vi "InitPos.vi"(8 "error in (no error)":errorcluster caption="错误输入（无错误）", 11 "RandomMoveBool 输入":refnum<class "RandomMoveBool.lvclass">) -> (0 "error out":errorcluster caption="错误输出", 3 "RandomMoveBool 输出":refnum<class "RandomMoveBool.lvclass">)   [LabVIEW 2018, in "RandomMoveBool.lvclass"]
uses:
  RandomMoveBool.lvclass
  <vilib>/Utility/miscctls.llb/LVPositionTypeDef.ctl
  RandomMoveBool.lvclass/RandomMoveBool.ctl
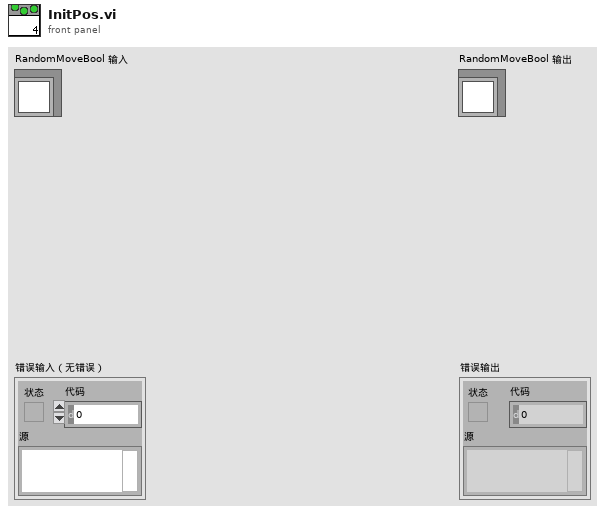
[diagram p1: front panel]
types:
  T1 = typedef "LVPositionTypeDef.ctl" = cluster{"Left":i32, "Top":i32}
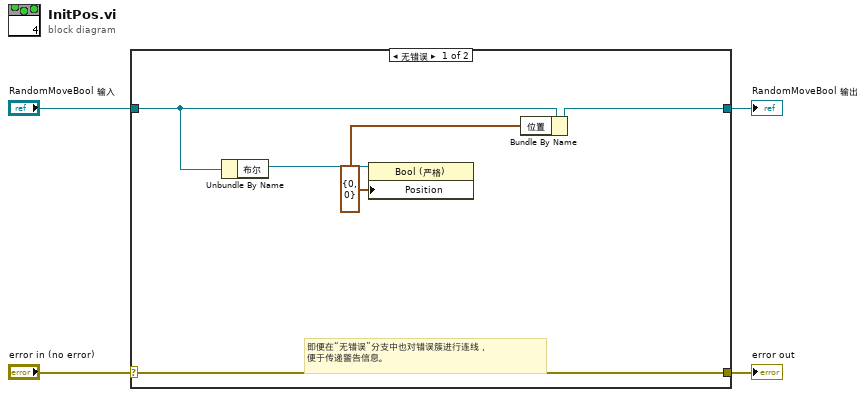
[diagram p0: block diagram]
diagram:
  n1 = case shown="无错误" "error in (no error)" {
    selector: "error in (no error)" -> [w9 w11]
    tunnel: [w9 w11] -> w3
    tunnel: [w6 w10] -> w1
    tunnel: "RandomMoveBool 输入" -> [w8 w10]
    frame No Error {
      w5 = T1 {"Left"=0, "Top"=0} ("位置")
      # "即便在“无错误”分支中也对错误簇进行连线，\n便于传递警告信息。"
      n2 = Unbundle By Name(w8) -> ("布尔"=w7:refnum<vi>)
      n3 = property class="Bool (严格)"(reference=w7, "Position"=w5) -> ()  [unwired: 1 in, 2 out]
      n4 = Bundle By Name(cluster=w8, "位置"=w5) -> (w6:refnum<class "RandomMoveBool.lvclass">)
    }
    frame Error {
    }
  }
  "error out" <- w3
  "RandomMoveBool 输出" <- w1
